vi "Acquire & Chart PointByPoint SynchroResolver.vi"() -> ()   [LabVIEW 8.6]
uses:
  vi.lib/UeiDaq/UeiDaqConfigureTimingForSimpleIO.vi
  vi.lib/UeiDaq/UeiDaqReadOneScaledScan.vi
  vi.lib/UeiDaq/UeiDaqCreateSynchroResolverSession.vi
  <libdir>/resource/objmgr/ueidaq.rc
panel:
  in  "Mode":enum16{"Synchro", "Resolver", "SynchroZGround"}(ring)
  in  "Excitation frequency":dbl
  in  "Excitation voltage":dbl
  in  "External Excitation":bool
  in  "timeout (ms)":u32
  in  "Resource":string
  out "Total scans acquired":i32
  out "Waveform Chart":dbl[][](graph)
  in  "Refresh rate (ms)":u32
  in  "stop":bool
  # "Software timed Synchro/Resolver measurement"
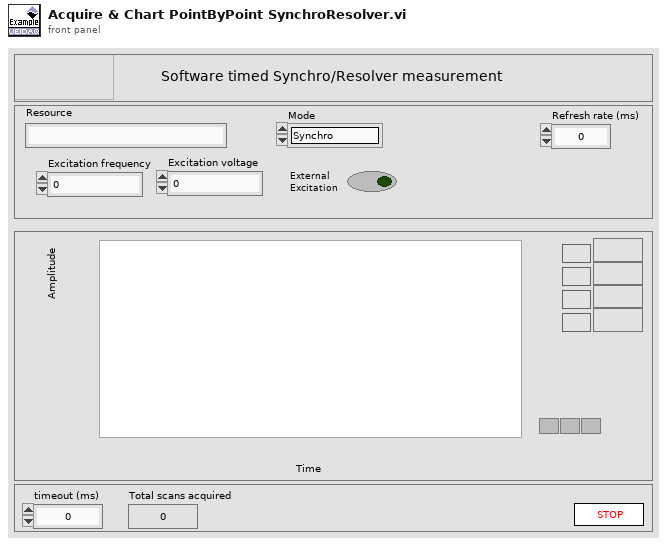
[diagram p1: front panel]
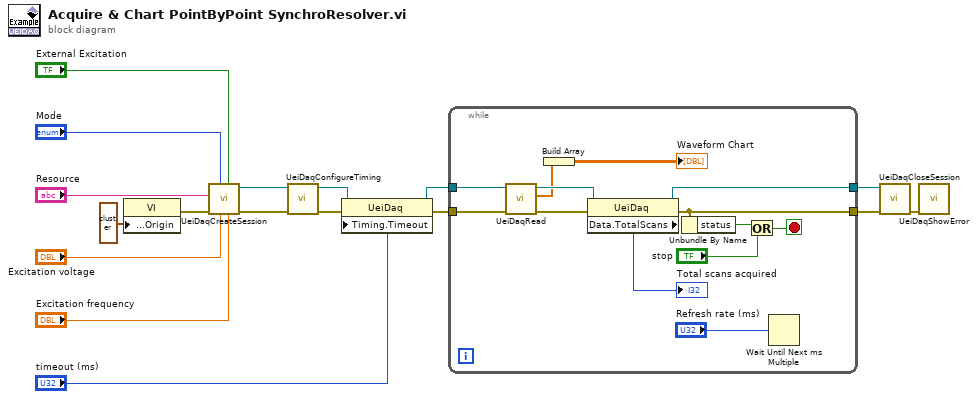
[diagram p0: block diagram]
diagram:
  n1 = property class="VI"("Front Panel.Origin"=cluster{"Horizontal":i16, "Vertical":i16} ? ("Front Panel Window:Origin")) -> (error out=w11:errorcluster)  [unwired: 2 in, 1 out]
  n2 = call-poly "UeiDaqCreateSession.vi"("Excitation frequency"="Excitation frequency", "External Excitation"="External Excitation", "Excitation voltage"="Excitation voltage", "Mode"="Mode", "error in (no error)"=w11, "Resource"="Resource") -> ("error out"=w2:errorcluster, "UeiDaq Refnum Out"=w14:refnum<k20>)  [unwired: 1 in, 3 out]
  n3 = call-poly "UeiDaqConfigureTiming.vi"("error in (no error)"=w2, "UeiDaq Refnum In"=w14) -> ("error out"=w10:errorcluster, "UeiDaq Refnum Out"=w8:refnum<k20>)  [unwired: 1 in, 7 out]
  n4 = property class="UeiDaq"(reference=w8, error in=w10, "Timing.Timeout"="timeout (ms)") -> (reference out=w7:refnum<k20>, error out=w9:errorcluster)
  n5 = while {
    tunnel: w7 -> [w26]
    tunnel: w9 -> [w27]
    tunnel: [w22] -> w15
    tunnel: [w21] -> w16
    stop <- w28 stop-if-true
    n6 = call-poly "UeiDaqRead.vi"("error in (no error)"=w27, "UeiDaq Refnum In"=w26) -> ("error out"=w23:errorcluster, "Scaled Data"=w19:dbl[], "UeiDaq Refnum Out"=w24:refnum<k20>)  [unwired: 7 out]
    n7 = Build Array(w19) -> (→"Waveform Chart":dbl[][])
    n8 = property class="UeiDaq"(reference=w24, error in=w23) -> (reference out=w21:refnum<k20>, error out=w22:errorcluster, "Data.TotalScans"=→"Total scans acquired":u32)
    n9 = Unbundle By Name(w22) -> ("status"=w30:bool)
    n10 = Or(x=w30, y="stop") -> (x .or. y?=w28:bool)
    n11 = Wait Until Next ms Multiple(millisecond multiple="Refresh rate (ms)") -> ()  [unwired: 1 out]
  }
  n12 = call "UeiDaqCloseSession.vi"("error in (no error)"=w15, "UeiDaq Refnum In"=w16) -> ("error out"=w17:errorcluster)  [unwired: 1 in, 8 out]
  n13 = call "UeiDaqShowError.vi"("error in (no error)"=w17) -> ()  [unwired: 2 in, 9 out]
